vi "CMSMismatch.vi"(1 "Conversion":T1, 3 "Input":dbl[](array[numeric])) -> (0 "Output":dbl[](array[numeric]))   [LabVIEW 2016]
uses:
  Remote VIs/Configs/CMSMismatch.ctl
  <userlib>/_OpenG.lib/array/array.llb/Index 1D Array Elements (DBL)__ogtk.vi
  <vilib>/NI/GXML/_subVIs/GXML SearchParser/Search Parser.vi
  <vilib>/NI/GXML/GXML.lvlib
panel:
  out "error out":errorcluster
  in  "error in (no error)":errorcluster
  in  "CMS File":path
  in  "Operation":enum16{"Init", "Convert"}(ring)
  out "SensorID":i32[](array[numeric])
  out "MotorID":i32[](array[numeric])
  out "CableID":i32[](array[numeric])
  out "Sensor0":dbl[](array[numeric])
  out "Motor0":dbl[](array[numeric])
  out "Cable0":dbl[](array[numeric])
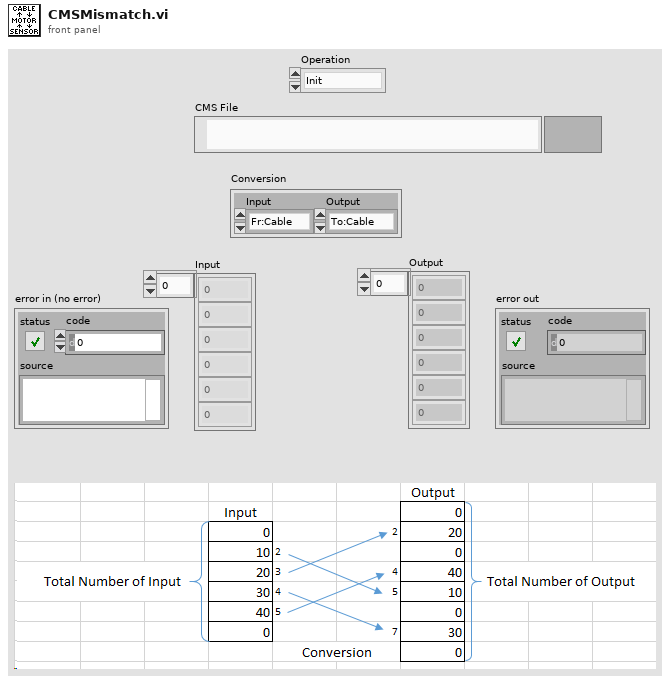
[diagram p1: front panel]
types:
  T1 = cluster{"Input":enum16{"Fr:Cable", "Fr:Motor", "Fr:Sensor"}, "Output":enum16{"To:Cable", "To:Motor", "To:Sensor"}}
  T2 = typedef "CMSMismatch.ctl" = cluster{"TotalCount":cluster{"CableCount":i32, "MotorCount":i32, "SensorCount":i32}, "Matches":cluster{"CableID":i32, "MotorID":i32, "SensorID":i32}[]}
  T3 = cluster{"CableCount":i32, "MotorCount":i32, "SensorCount":i32}
  T4 = cluster{"CableID":i32, "MotorID":i32, "SensorID":i32}[]
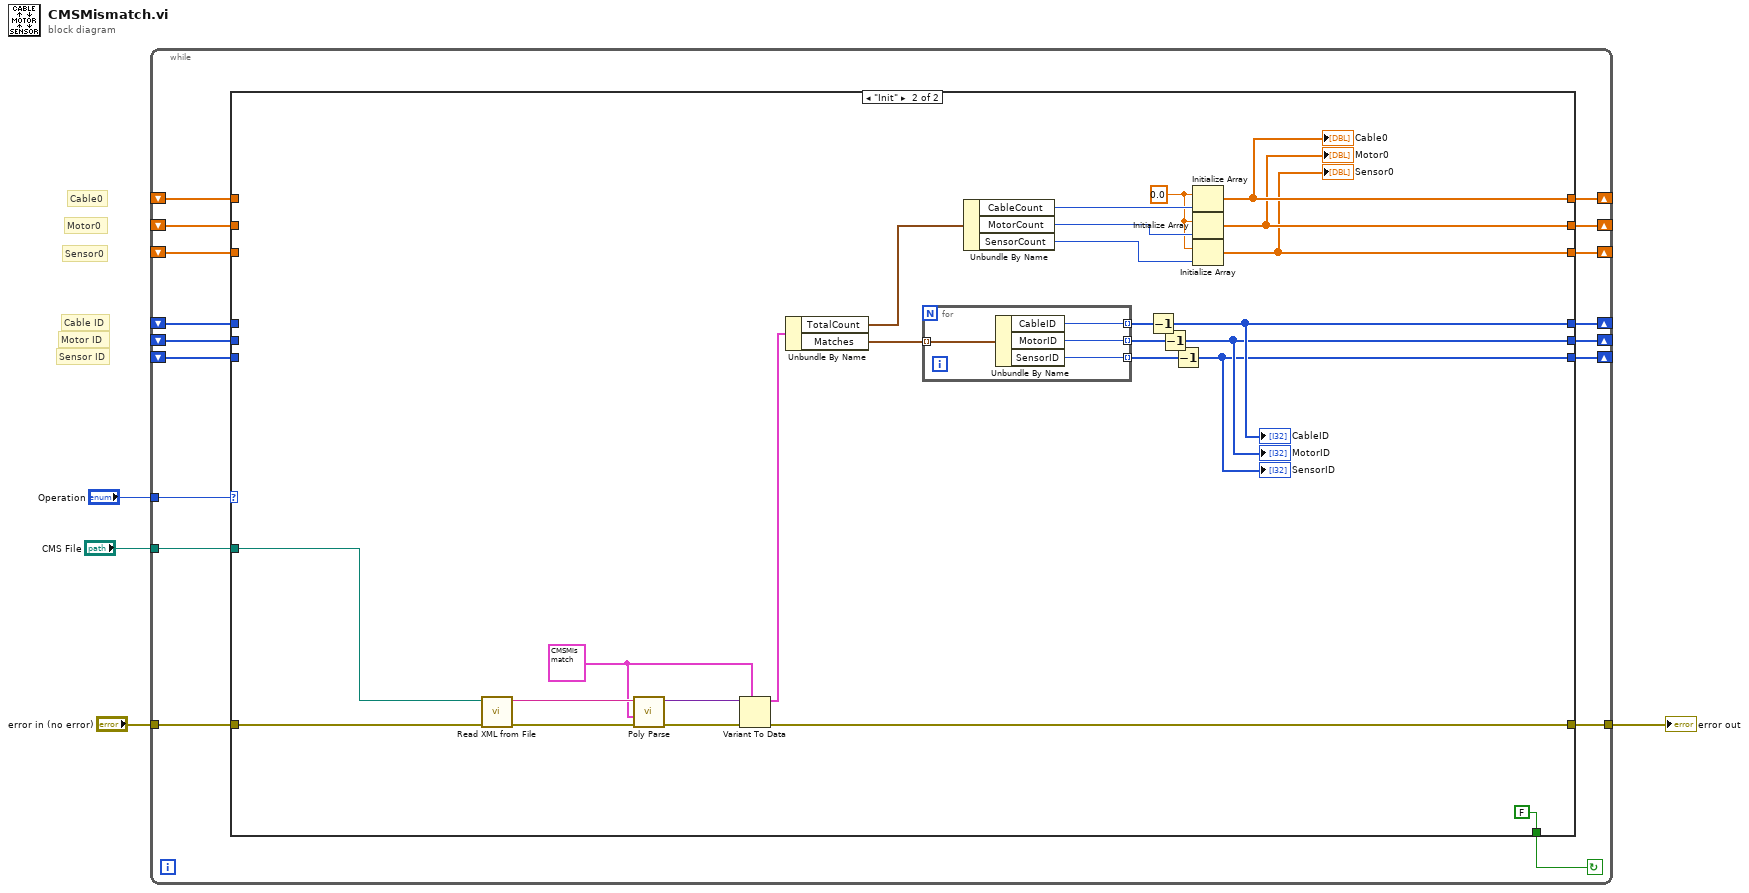
[diagram p0: block diagram]
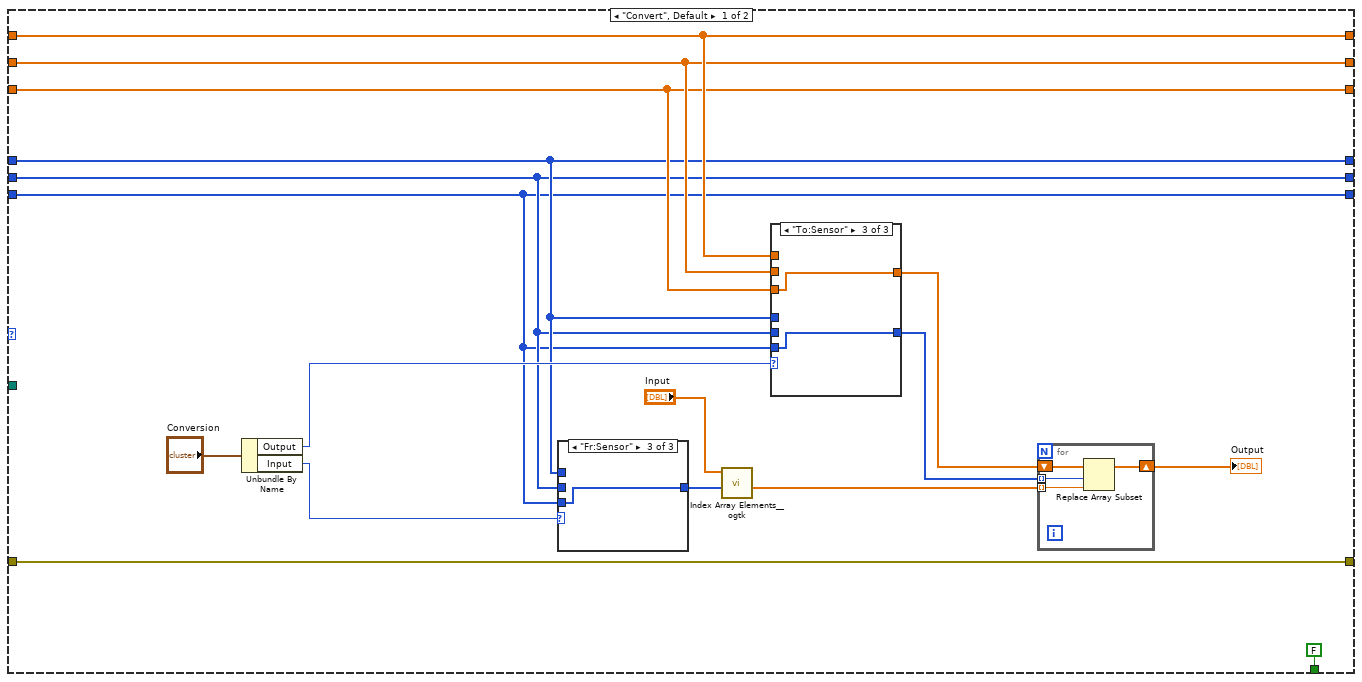
[diagram p2: hidden frame]
diagram:
  # "Sensor ID"
  # "Motor ID"
  # "Cable ID"
  # "Sensor0"
  # "Motor0"
  # "Cable0"
  n1 = while {
    shift-right: [w21] -> _
    shift-left: _ -> [w15]
    shift-right: [w20] -> _
    shift-left: _ -> [w14]
    shift-right: [w19] -> _
    shift-left: _ -> [w13]
    shift-right: [w18] -> _
    shift-left: _ -> [w12]
    shift-right: [w17] -> _
    shift-left: _ -> [w11]
    shift-right: [w16] -> _
    shift-left: _ -> [w10]
    tunnel: "Operation" -> [w8]
    tunnel: "CMS File" -> [w7]
    tunnel: "error in (no error)" -> [w6]
    tunnel: [w5] -> w1
    stop <- w9 continue-if-true
    n2 = case shown="\"Init\"" w8 {
      tunnel: [w32 w76] -> w21
      tunnel: [w31 w75] -> w20
      tunnel: [w30 w74] -> w19
      tunnel: [w29 w73] -> w18
      tunnel: [w28 w72] -> w17
      tunnel: [w27 w71] -> w16
      tunnel: w15 -> [w32 _]
      tunnel: w14 -> [w31 _]
      tunnel: w13 -> [w30 _]
      tunnel: w12 -> [w29 _]
      tunnel: w11 -> [w28 _]
      tunnel: w10 -> [w27 _]
      tunnel: [FALSE FALSE] -> w9
      tunnel: w7 -> [_ w62]
      tunnel: w6 -> [w22 w61]
      tunnel: [w22 w56] -> w5
      frame "Convert", Default {
        n3 = Unbundle By Name("Conversion") -> ("Output"=w33:enum16{"To:Cable", "To:Motor", "To:Sensor"}, "Input"=w34:enum16{"Fr:Cable", "Fr:Motor", "Fr:Sensor"})
        n4 = case shown="\"Fr:Sensor\"" w34 {
          tunnel: w29 -> [w45 _ _]
          tunnel: w28 -> [_ w46 _]
          tunnel: w27 -> [_ _ w47]
          tunnel: [w45 w46 w47] -> w37
          frame "Fr:Cable" {
          }
          frame "Fr:Motor" {
          }
          frame "Fr:Sensor" {
          }
        }
        n5 = call-poly <userlib>:"Index Array Elements__ogtk.vi"("indices"=w37, "array"="Input") -> ("elements"=w38:dbl[])  [unwired: 9 in]
        n6 = case shown="\"To:Sensor\"" w33 {
          tunnel: w29 -> [w40 _ _]
          tunnel: w28 -> [_ w42 _]
          tunnel: w27 -> [_ _ w44]
          tunnel: [w40 w42 w44] -> w35
          tunnel: w32 -> [w39 _ _]
          tunnel: w31 -> [_ w41 _]
          tunnel: w30 -> [_ _ w43]
          tunnel: [w39 w41 w43] -> w36
          frame "To:Cable" {
          }
          frame "To:Motor" {
          }
          frame "To:Sensor" {
          }
        }
        n7 = for {
          tunnel: w35 -> [w50] mode=indexing
          tunnel: w38 -> [w49] mode=indexing
          shift-right: [w48] -> w25
          shift-left: w36 -> [w51]
          n8 = Replace Array Subset(array=w51, new element=w49, index=w50) -> (w48:dbl[])
        }
        "Output" <- w25
      }
      frame "Init" {
        w52 = T2 {"TotalCount"={"CableCount"=0, "MotorCount"=0, "SensorCount"=0}, "Matches"=[{"CableID"=4, "MotorID"=8, "SensorID"=8}, {"CableID"=1, "MotorID"=6, "SensorID"=8}, {"CableID"=2, "MotorID"=5, "SensorID"=5}, {"CableID"=3, "MotorID"=7, "SensorID"=4}, {"CableID"=4, "MotorID"=4, "SensorID"=2}]} ("CableMotorSensorMismatch")
        w67 = 0.0 ("element")
        n9 = call <vilib>:"Read XML from File.vi"("error in"=w61, "XML File Path"=w62) -> ("error out"=w60:errorcluster, "XML String Out"=w59:string)  [unwired: 8 in]
        n10 = call-poly <vilib>:"Poly Parse.vi"("error in"=w60, "TypeDesc"=w52, "XML String In"=w59) -> ("error out"=w57:errorcluster, "Parsed Data"=w58:variant)  [unwired: 7 in]
        n11 = Variant To Data(error in=w57, type=w52, Variant=w58) -> (data=w55:T2, error out=w56:errorcluster)
        n12 = Unbundle By Name(w55) -> ("TotalCount"=w53:T3, "Matches"=w54:T4)
        n13 = for {
          tunnel: w54 -> [w80] mode=indexing
          tunnel: [w79] -> w64 mode=indexing
          tunnel: [w78] -> w66 mode=indexing
          tunnel: [w77] -> w65 mode=indexing
          n14 = Unbundle By Name(w80) -> ("CableID"=w79:i32, "MotorID"=w78:i32, "SensorID"=w77:i32)
        }
        n15 = Unbundle By Name(w53) -> ("CableCount"=w70:i32, "MotorCount"=w69:i32, "SensorCount"=w68:i32)
        n16 = Decrement(x=w64) -> (x-1=w73:i32[])
        "CableID" <- w73
        n17 = Decrement(x=w66) -> (x-1=w72:i32[])
        "MotorID" <- w72
        n18 = Decrement(x=w65) -> (x-1=w71:i32[])
        "SensorID" <- w71
        n19 = Initialize Array(w67, w70) -> (w76:dbl[])
        "Cable0" <- w76
        n20 = Initialize Array(w67, w69) -> (w75:dbl[])
        "Motor0" <- w75
        n21 = Initialize Array(w67, w68) -> (w74:dbl[])
        "Sensor0" <- w74
      }
    }
  }
  "error out" <- w1
